vi "Shared_Relay_ConnectDisconnect.vi"(7 "Relay Action":T1=21 items=["Open Relay"=20, "Close Relay"=21], 10 "Relays":tag[](array[tag]), 11 "Semiconductor Module Context":T2) -> (0 "error Out":errorcluster)   [LabVIEW 2020, in "Shared.lvlib"]
doc: "Connect / Disconnect Relay Driver channels"
uses:
  Shared.lvlib
  <vilib>/NI_TestStand_SemiconductorModule/NI_TestStand_Semiconductor_Module.lvlibp/PinMap/General/SemiconductorModuleContext.ctl
  <instrlib>/niSwitch/niSwitch.llb/niSwitch Relay Action.ctl
  <vilib>/NI_TestStand_SemiconductorModule/NI_TestStand_Semiconductor_Module.lvlibp/PinMap/Relay Driver/RelaysToRelayDriverNISWITCHSessions.vi
  <vilib>/NI_TestStand_SemiconductorModule/NI_TestStand_Semiconductor_Module.lvlibp
  ResourceHandling/ResourceHandling.lvlib
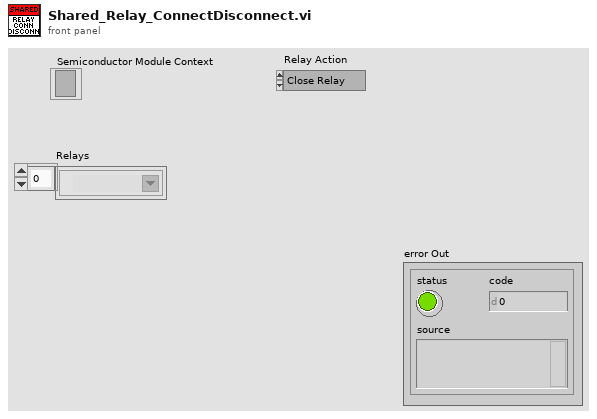
[diagram p1: front panel]
types:
  T1 = typedef "niSwitch Relay Action.ctl" = i32
  T2 = typedef "NI_TestStand_Semiconductor_Module.lvlibp/SemiconductorModuleContext.ctl" = refnum<k7>
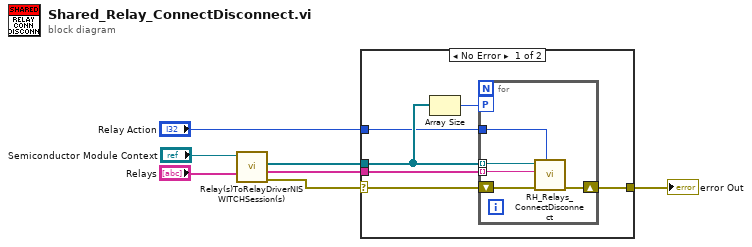
[diagram p0: block diagram]
diagram:
  n1 = call-poly <vilib>:"Relay(s)ToRelayDriverNISWITCHSession(s).vi"("Relays"="Relays", "Semiconductor Module Context"="Semiconductor Module Context") -> ("error out"=w4:errorcluster, "NI-SWITCH Relay Names"=w2:string[], "NI-SWITCH Sessions"=w3:refnum<k15>[])  [unwired: 6 in, 1 out]
  n2 = case shown="No Error" w4 {
    selector: w4 -> [w11 w19]
    tunnel: [w12 w19] -> w7
    tunnel: w3 -> [w9 _]
    tunnel: w2 -> [w10 _]
    tunnel: "Relay Action" -> [w8 _]
    frame No Error {
      n3 = Array Size(array=w9) -> (size(s)=w13:i32)
      n4 = for {
        workers-P: w13 -> [_]
        shift-right: [w15] -> w12
        shift-left: w11 -> [w17]
        tunnel: w9 -> [w18] mode=indexing
        tunnel: w10 -> [w16] mode=indexing
        tunnel: w8 -> [w14]
        n5 = call "RH_Relays_ConnectDisconnect.vi"("relay action (Close Relay)"=w14, "error in"=w17, "relay names"=w16, "Relays Session In"=w18) -> ("error out"=w15:errorcluster)  [unwired: 6 in, 1 out]
      }
    }
    frame Error {
    }
  }
  "error Out" <- w7
